vi "PH_BackreflectionMeas.get data to modify.vi"(0 "i ref in":refnum<vi>, 3 "ms timeout (10000)":i32=10000, 5 "error in (no error)":errorcluster) -> (14 "i ref out":refnum<vi>, 16 "i attribute":T1={"GUI Refs"={"Get Data"=refnum, "BR State"=refnum, "Reset warning"=refnum, "Low Energy Graph"=refnum}, "Status"={"Reset Warning"=FALSE}, "Default Low Energy Chan Settings"={"Channel Name"="CH1", "Input Impedance"="MEG", "Max Input Frequency"="TWENTY", "Vertical Coupling"=1, "Channel Enabled"=TRUE, "Probe Attenuation"=1.0, "Vertical Range"=100.0, "Vertical Offset"=0.0}, "Default High Energy Chan Settings"={"Channel Name"="CH1", "Input Impedance"="MEG", "Max Input Frequency"="TWENTY", "Vertical Coupling"=1, "Channel Enabled"=TRUE, "Probe Attenuation"=1.0, "Vertical Range"=100.0, "Vertical Offset"=0.0}, "Default Trigger Settings"={"Source"="CH1", "Slope"=0, "Level [V]"=0.0}, "Default Acqu Settings"={"Time base"=2e-07, "Record Length"=10000, "Start Time"=0.0, "Type"=0, "Continuous"=FALSE}, "Limit [V]"=0.0} {"Default Acqu Settings"."Start Time" format="%#_12p"; "Default Acqu Settings"."Record Length" items=["500"=500, "10000"=10000]; "Default Acqu Settings"."Time base" items=["2ns"=2e-09, "4ns"=4e-09, "10ns"=1e-08, "20ns"=2e-08, "40ns"=4e-08, "100ns"=1e-07, "200ns"=2e-07, "400ns"=4e-07, "1µs"=1e-06, "2µs"=2e-06, "4µs"=4e-06, "10µs"=1e-05, "20µs"=2e-05, "40µs"=4e-05, "100µs"=0.0001, "200µs"=0.0002, "400µs"=0.0004, "1ms"=0.001, "2ms"=0.002, "10ms"=0.01, "20ms"=0.02, "40ms"=0.04, "100ms"=0.1, "200ms"=0.2, "400ms"=0.4, "1s"=1.0, "2s"=2.0, "4s"=4.0, "10s"=10.0]; "Default Trigger Settings"."Level [V]" format="%#_6p"; "Default High Energy Chan Settings"."Vertical Offset" format="%#_6p"; "Default High Energy Chan Settings"."Vertical Range" items=["1mV"=0.001, "2mV"=0.002, "5mV"=0.005, "10mV"=0.01, "20mV"=0.02, "50mV"=0.05, "100mV"=0.1, "200mV"=0.2, "500mV"=0.5, "1V"=1.0]; "Default High Energy Chan Settings"."Probe Attenuation" format="%#.2f"; "Default Low Energy Chan Settings"."Vertical Offset" format="%#_6p"; "Default Low Energy Chan Settings"."Vertical Range" items=["1mV"=0.001, "2mV"=0.002, "5mV"=0.005, "10mV"=0.01, "20mV"=0.02, "50mV"=0.05, "100mV"=0.1, "200mV"=0.2, "500mV"=0.5, "1V"=1.0]; "Default Low Energy Chan Settings"."Probe Attenuation" format="%#.2f"}, 17 "timed out":bool, 19 "error out":errorcluster)   [LabVIEW 2014, in "PH_BackreflectionMeas.lvlib"]
doc: "Reads the attribute data of the object after the access to the data has been locked by the \"acquire\" method. If the attribute data has been locked already, this methods waits until the attribute data is unlocked or there is a timeout.\n\nThe attribute data must be unlocked using the methods \"release\" or \"set modified data\".\n\nLicense Agreement for this software:\n\nCopyright (C)\nGesellschaft für Schwerionenforschung, GSI\nPlanckstr. 1\n64291 Darmstadt\nGermany\n\nContact: D.Beck@gsi.de \n\nThis program is free software; you can redistribute it and/or modify it under the terms of the GNU General Public License as published by the Free Software Foundation; either version 2 of the license, or (at your option) any later version.\n\nThis program is distributed in the hope that it will be useful, but WITHOUT ANY WARRANTY; without even the implied warranty of MERCHANTABILITY or FITNESS FOR A PARTICULAR PURPOSE. See the GNU General License for more details (http://www.gnu.org).\n\nGesellschaft für Schwerionenforschung, GSI\nPlanckstr. 1, 64291 Darmstadt, Germany\nFor all questions and ideas contact: M.Richter@gsi.de, H.Brand@gsi.de or D.Beck@gsi.de.\nLast update: 17-JUN-2004"
uses:
  PH_BackreflectionMeas.lvlib
  PH_BackreflectionMeas.i attribute.ctl
  PH_Devices/PH_TKTDS-30xx/PH_TKTDS-30xx.Channel Config.ctl
  PH_Devices/PH_TKTDS-30xx/PH_TKTDS-30xx.Trigger Config.ctl
  PH_Devices/PH_TKTDS-30xx/PH_TKTDS-30xx.Acquisition Config.ctl
  CS_Core/CSObj/CSObj.lvlib
  PH_Devices/PH_TKTDS-30xx/PH_TKTDS-30xx.lvlib
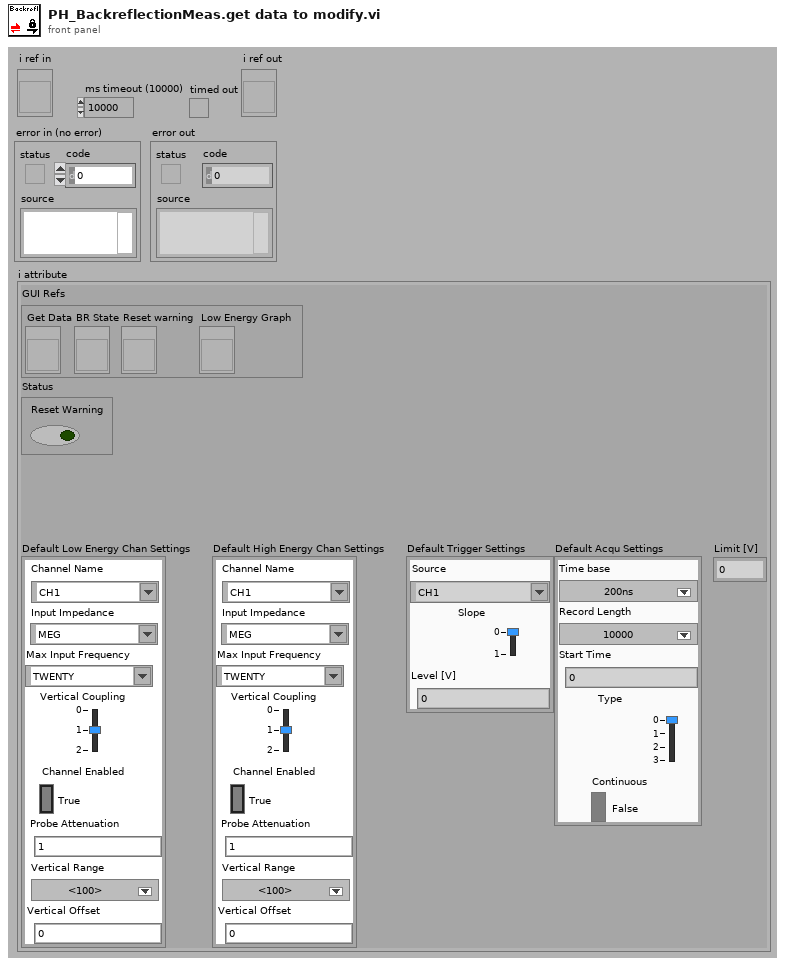
[diagram p1: front panel]
types:
  T1 = typedef "PH_BackreflectionMeas.lvlib/PH_BackreflectionMeas.i attribute.ctl" = cluster{"GUI Refs":cluster{"Get Data":refnum<vi>, "BR State":refnum<vi>, "Reset warning":refnum<vi>, "Low Energy Graph":refnum<vi>}, "Status":cluster{"Reset Warning":bool}, "Default Low Energy Chan Settings":T2, "Default High Energy Chan Settings":T2, "Default Trigger Settings":T3, "Default Acqu Settings":T4, "Limit [V]":dbl}
  T2 = typedef "PH_TKTDS-30xx.lvlib/PH_TKTDS-30xx.Channel Config.ctl" = cluster{"Channel Name":string, "Input Impedance":string, "Max Input Frequency":string, "Vertical Coupling":i32, "Channel Enabled":bool, "Probe Attenuation":dbl, "Vertical Range":dbl, "Vertical Offset":dbl}
  T3 = typedef "PH_TKTDS-30xx.lvlib/PH_TKTDS-30xx.Trigger Config.ctl" = cluster{"Source":string, "Slope":i32, "Level [V]":dbl}
  T4 = typedef "PH_TKTDS-30xx.lvlib/PH_TKTDS-30xx.Acquisition Config.ctl" = cluster{"Time base":dbl, "Record Length":u16, "Start Time":dbl, "Type":i32, "Continuous":bool}
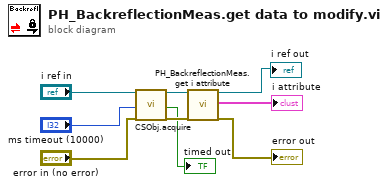
[diagram p0: block diagram]
diagram:
  n1 = call "CSObj.acquire.vi"("i ref in"="i ref in", "ms timeout (10000)"="ms timeout (10000)", "error in (no error)"="error in (no error)") -> ("i ref out"=w8:refnum<vi>, "timed out"=→"timed out":bool, "error out"=w5:errorcluster)  [unwired: 14 in]
  n2 = call "PH_BackreflectionMeas.get i attribute.vi"("i ref in"=w8, "error in (no error)"=w5) -> ("i ref out"=→"i ref out":refnum<vi>, "i attribute"=→"i attribute":T1, "error out"=→"error out":errorcluster)  [unwired: 15 in]
